vi "INIT HP Freq.vi"   [LabVIEW 2019]
uses:
  MWC Global.vi
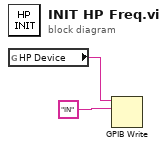
[diagram p0: block diagram]
diagram:
  n1 = global read "MWC Global.vi" "HP Device"() -> (w1:string)
  n2 = GPIB Write(0:w1, 1:"IN" ("data")) -> ()  [unwired: 3 in, 2 out]
